vi "Q_kulso.vi"(5 "idolepes":dbl=1.0, 6 "F_10_11":dbl, 7 "F_kulso_levego_fal":dbl, 9 "F_kulso_vektor":dbl[](array[numeric]), 10 "Q_kulso_elozo_vektor":dbl[](array[numeric])) -> (2 "Q_kulso_aktualis_vektor":dbl[](array[numeric]))   [LabVIEW 2013]
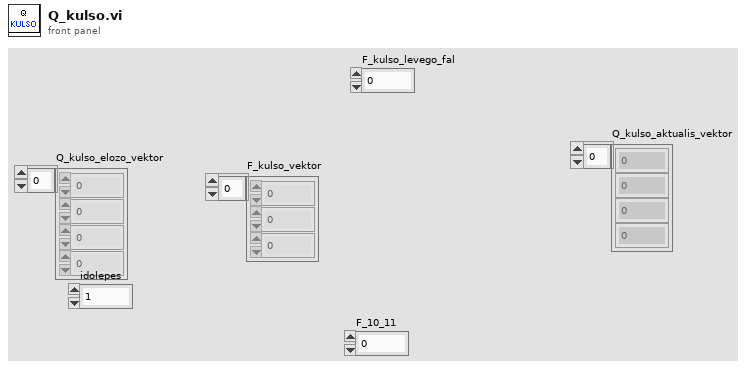
[diagram p1: front panel]
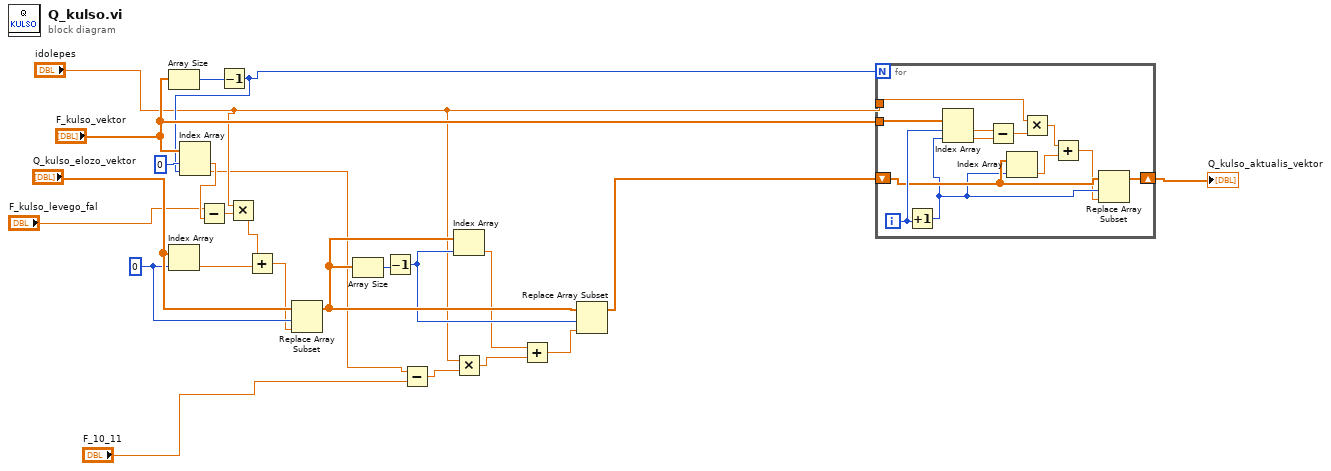
[diagram p0: block diagram]
diagram:
  w14 = 0 ("index")
  n1 = Array Size(array="F_kulso_vektor") -> (size(s)=w21:i32)
  n2 = Index Array(array="Q_kulso_elozo_vektor", index=w14) -> (element=w19:dbl)
  n3 = Decrement(x=w21) -> (x-1=w20:i32)
  n4 = Index Array(array="F_kulso_vektor", index #1=0 ("index"), index #2=w20) -> (element #1=w18:dbl, element #2=w3:dbl)
  n5 = Subtract(x="F_kulso_levego_fal", y=w18) -> (x-y=w17:dbl)
  n6 = Multiply(x="idolepes", y=w17) -> (x*y=w16:dbl)
  n7 = Add(x=w16, y=w19) -> (x+y=w13:dbl)
  n8 = Replace Array Subset(array="Q_kulso_elozo_vektor", new element=w13, index=w14) -> (w11:dbl[])
  n9 = Array Size(array=w11) -> (size(s)=w10:i32)
  n10 = Decrement(x=w10) -> (x-1=w9:i32)
  n11 = Subtract(x=w3, y="F_10_11") -> (x-y=w4:dbl)
  n12 = Index Array(array=w11, index=w9) -> (element=w7:dbl)
  n13 = Multiply(x="idolepes", y=w4) -> (x*y=w6:dbl)
  n14 = Add(x=w7, y=w6) -> (x+y=w8:dbl)
  n15 = Replace Array Subset(array=w11, new element=w8, index=w9) -> (w12:dbl[])
  n16 = for {
    N: w20 -> [_]
    tunnel: "F_kulso_vektor" -> [w36]
    tunnel: "idolepes" -> [w31]
    shift-right: [w25] -> w24
    shift-left: w12 -> [w30]
    i -> [w35]
    n17 = Increment(x=w35) -> (x+1=w29:i32)
    n18 = Index Array(array=w36, index #1=w35, index #2=w29) -> (element #1=w33:dbl, element #2=w34:dbl)
    n19 = Subtract(x=w33, y=w34) -> (x-y=w32:dbl)
    n20 = Index Array(array=w30, index=w29) -> (element=w27:dbl)
    n21 = Multiply(x=w31, y=w32) -> (x*y=w28:dbl)
    n22 = Add(x=w28, y=w27) -> (x+y=w26:dbl)
    n23 = Replace Array Subset(array=w30, new element=w26, index=w29) -> (w25:dbl[])
  }
  "Q_kulso_aktualis_vektor" <- w24
